vi "Pump Status.vi"() -> ()   [LabVIEW 2021]
uses:
  Controls/Pump Feeder.ctl
panel:
  out "Pump Status":T1
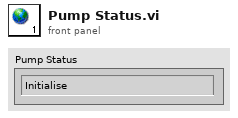
[diagram p1: front panel]
types:
  T1 = typedef "Pump Feeder.ctl" = enum16{"Initialise", "Waiting For Pumps 1", "Gate Open", "Wait for Delay", "Gate Close", "Waiting For Pumps 2", "Done", "Error"}
diagram:
